vi "MPX Check Sequence.vi"(8 "error in":errorcluster, 11 "sequence in":T1(array[cluster]) caption="Sequence definition" {"Channel" items=["A", "B"]}) -> (0 "error out":errorcluster, 3 "sequence out":T1(array[cluster]) caption="Sequence definition" {"Channel" items=["A", "B"]})   [LabVIEW 2013]
doc: "Checks multiplexer sequence for error."
uses:
  <vilib>/Utility/error.llb/Error Cluster From Error Code.vi
  <vilib>/ErrorRing/Error Ring.xnode
panel:
  out "sequence items":u16[](array[numeric])
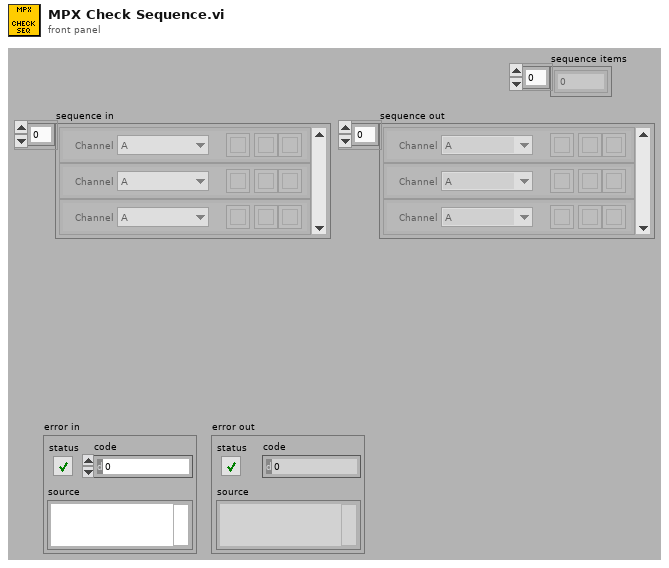
[diagram p1: front panel]
types:
  T1 = cluster{"btn clr":bool, "btn up":bool, "btn down":bool, "Channel":u16}[]
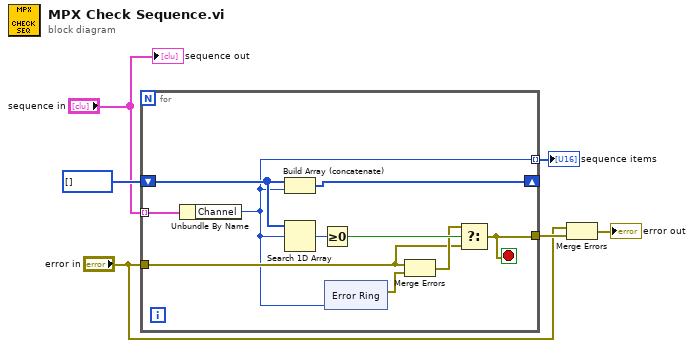
[diagram p0: block diagram]
diagram:
  n1 = for {
    tunnel: "sequence in" -> [w16] mode=indexing
    shift-right: [w9] -> _
    shift-left: i32[] [] -> [w15]
    tunnel: "error in" -> [w10]
    tunnel: [w8] -> w5
    tunnel: [w7] -> w1 mode=indexing
    stop <- w8 stop-if-true
    n2 = Unbundle By Name(w16) -> ("Channel"=w7:u16)
    n3 = Build Array (concatenate)(w15, w7) -> (w9:i32[])
    n4 = Search 1D Array(1D array=w15, element=w7) -> (index of element=w14:i32)  [unwired: 1 in]
    n5 = Greater Or Equal To 0?(x=w14) -> (x >= 0?=w13:bool)
    n6 = xnode "Error Ring"("parameter 0"=w7) -> ("error out"=w11:errorcluster)
    n7 = Merge Errors(w10, w11) -> (w12:errorcluster)
    n8 = Select(t=w12, s=w13, f=w10) -> (s? t:f=w8:errorcluster)
  }
  "sequence items" <- w1
  n9 = Merge Errors("error in", w5) -> (→"error out":errorcluster)
  "sequence out" <- "sequence in"
